vi "VALVE_calculate_valve_position.vi"(2 "valve positions":cluster{"Valve H":u8, "OldVal":u8}) -> (0 "Valves positions Old":u8[](array[numeric]), 1 "Valves positions New":u8[](array[numeric]))   [LabVIEW 2015]
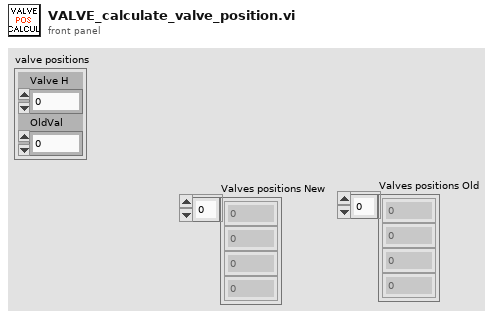
[diagram p1: front panel]
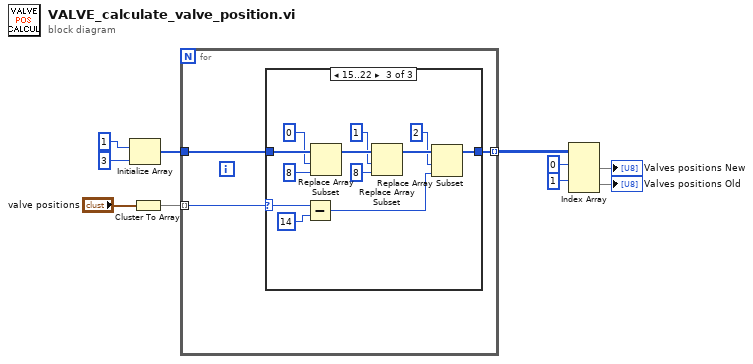
[diagram p0: block diagram]
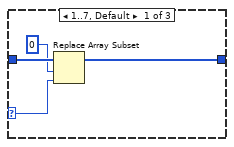
[diagram p2: hidden frame]
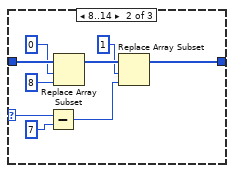
[diagram p3: hidden frame]
diagram:
  n1 = Initialize Array(u8 1 ("element"), 3 ("dimension size")) -> (w6:u8[])
  n2 = Cluster To Array(cluster="valve positions") -> (array=w9:u8[])
  n3 = for {
    tunnel: w9 -> [w11] mode=indexing
    tunnel: w6 -> [w13]
    tunnel: [w12] -> w5 mode=indexing
    n4 = case shown="15..22" w11 {
      selector: w11 -> [w14 w20 w29]
      tunnel: w13 -> [w17 w26 w38]
      tunnel: [w15 w22 w31] -> w12
      frame 1..7, Default {
        n5 = Replace Array Subset(array=w17, new element=w14, index=0 ("disabled index (row)")) -> (w15:u8[])
      }
      frame 8..14 {
        n6 = Subtract(x=w20, y=u8 7) -> (x-y=w18:u8)
        n7 = Replace Array Subset(array=w26, new element=u8 8 ("new element/subarray"), index=0 ("disabled index (row)")) -> (w23:u8[])
        n8 = Replace Array Subset(array=w23, new element=w18, index=1) -> (w22:u8[])
      }
      frame 15..22 {
        n9 = Subtract(x=w29, y=u8 14) -> (x-y=w27:u8)
        n10 = Replace Array Subset(array=w38, new element=u8 8 ("new element/subarray"), index=0 ("disabled index (row)")) -> (w35:u8[])
        n11 = Replace Array Subset(array=w35, new element=u8 8 ("new element/subarray"), index=1) -> (w32:u8[])
        n12 = Replace Array Subset(array=w32, new element=w27, index=2) -> (w31:u8[])
      }
    }
  }
  n13 = Index Array(array=w5, index (row) #1=0 ("index (row)"), index (row) #2=1 ("index (row)")) -> (element #1=→"Valves positions New":u8[], element #2=→"Valves positions Old":u8[])  [unwired: 2 in]
